vi "HC MFR loff.vi"(7 "Flow rate":dbl, 8 "O2 Eq Up":dbl, 9 "O2 Measured":dbl, 10 "O2t %":dbl, 11 "Lambda_t":dbl) -> (3 "HC MFR":dbl)   [LabVIEW 2014]
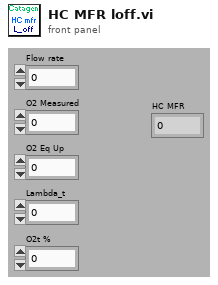
[diagram p1: front panel]
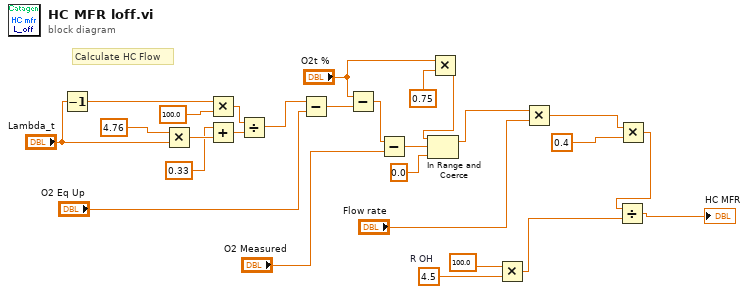
[diagram p0: block diagram]
diagram:
  w18 = 4.5  # R OH
  # "Calculate HC Flow"
  n1 = Decrement(x="Lambda_t") -> (x-1=w27:dbl)
  n2 = Multiply(x=4.76, y="Lambda_t") -> (x*y=w24:dbl)
  n3 = Multiply(x=w27, y=100.0) -> (x*y=w25:dbl)
  n4 = Add(x=0.33, y=w24) -> (x+y=w23:dbl)
  n5 = Divide(x=w25, y=w23) -> (x/y=w7:dbl)
  n6 = Subtract(x=w7, y="O2 Eq Up") -> (x-y=w5:dbl)
  n7 = Subtract(x="O2t %", y=w5) -> (x-y=w4:dbl)
  n8 = Subtract(x=w4, y="O2 Measured") -> (x-y=w14:dbl)
  n9 = Multiply(x="O2t %", y=0.75) -> (x*y=w10:dbl)
  n10 = In Range and Coerce(upper limit=w10, x=w14, lower limit=0.0) -> (coerced(x)=w13:dbl)  [unwired: 1 out]
  n11 = Multiply(x=100.0 ("y"), y=w18) -> (x*y=w17:dbl)
  n12 = Multiply(x=w13, y="Flow rate") -> (x*y=w2:dbl)
  n13 = Multiply(x=w2, y=0.4) -> (x*y=w1:dbl)
  n14 = Divide(x=w1, y=w17) -> (x/y=→"HC MFR":dbl)
